vi "Test_Attribute.vi"() -> ()   [LabVIEW 2013]
uses:
  source/Serializer.INI/Serializer.PlainText.INI.lvclass
  source/Serializer/Serializer.lvclass
panel:
  out "String-formatted Value 2":string
  out "String-formatted Value":string
  out "String":string
  out "data":T1
  out "error out":errorcluster
  out "Section Attributes":variant
  out "Value":variant
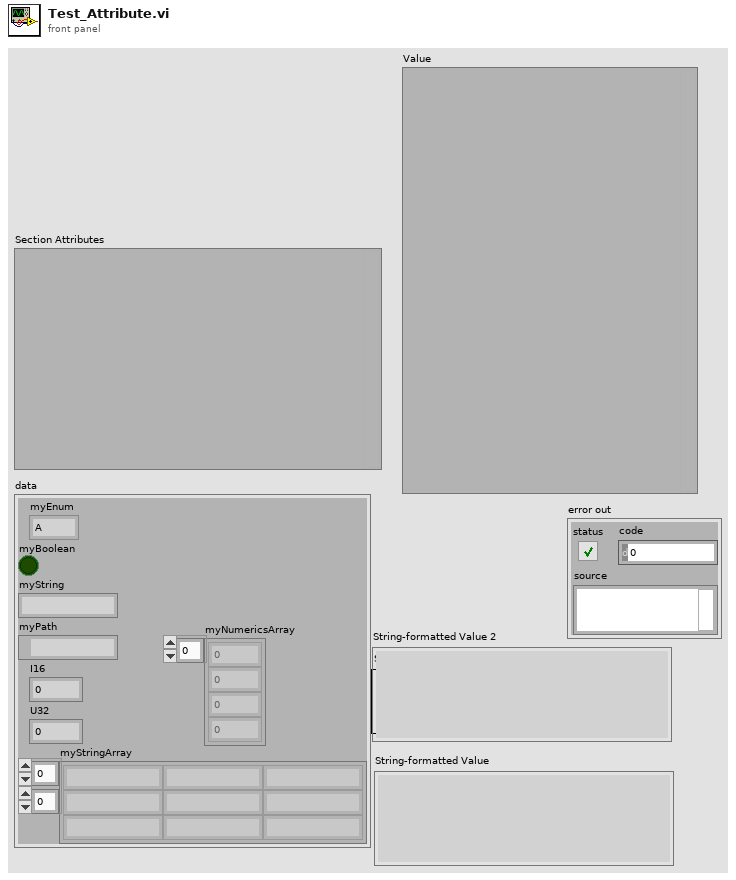
[diagram p1: front panel]
types:
  T1 = cluster{"myEnum":enum16{"A", "B", "C", "D"}, "myBoolean":bool, "myString":string, "myPath":path, "I16":i16, "U32":cdb, "myStringArray":string[][], "myNumericsArray":dbl[]}
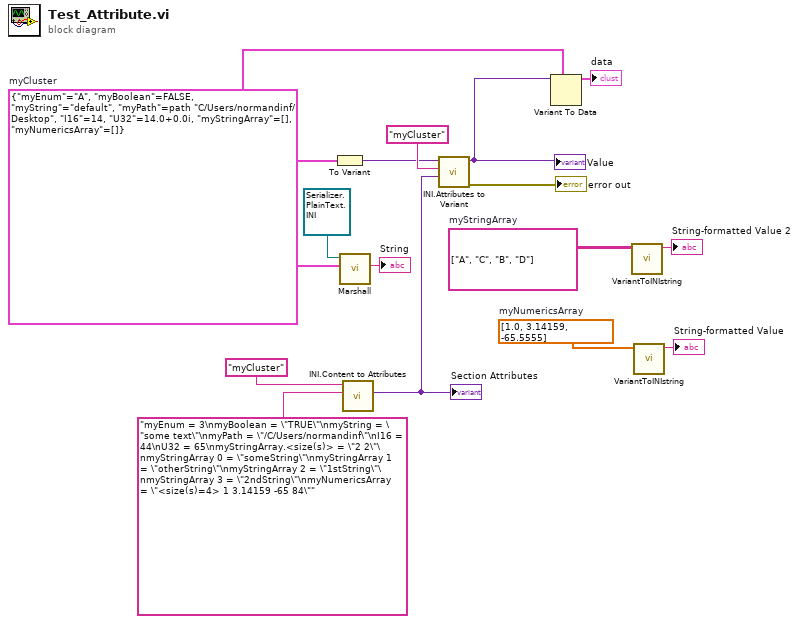
[diagram p0: block diagram]
diagram:
  w1 = string[][] [["A", "C"], ["B", "D"]]  # myStringArray
  w4 = dbl[] [1.0, 3.14159, -65.5555]  # myNumericsArray
  w6 = T1 {"myEnum"=enum."A", "myBoolean"=FALSE, "myString"="default", "myPath"=path "C:/Users/normandinf/Desktop", "I16"=14, "U32"=14.0+0.0i, "myStringArray"=[], "myNumericsArray"=[]}  # myCluster
  n1 = To Variant(anything=w6) -> (Variant=w11:variant)
  n2 = call "Marshall.vi"("Variant"=w6, "Serializer in"=refnum<class "Serializer.PlainText.INI.lvclass"> refnum ("Serializer.PlainText.INI.lvclass")) -> ("String"=→"String":string)  [unwired: 7 in, 2 out]
  n3 = call "INI.Content to Attributes.vi"("Content"="myEnum = 3\nmyBoolean = \"TRUE\"\nmyString = \"some text\"\nmyPath = \"/C/Users/normandinf\"\nI16 = 44\nU32 = 65\nmyStringArray.<size(s)> = \"2 2\"\nmyStringArray 0 = \"someString\"\nmyStringArray 1 = \"otherString\"\nmyStringArray 2 = \"1stString\"\nmyStringArray 3 = \"2ndString\"\nmyNumericsArray = \"<size(s)=4> 1 3.14159 -65 84\"", "Section Name"="myCluster" ("Content")) -> ("Section Attributes"=w15:variant)  [unwired: 9 in]
  "Section Attributes" <- w15
  n4 = call "INI.Attributes to Variant.vi"("Section Attribute"=w15, "Data Name"="myCluster" ("Content"), "Datatype"=w11) -> ("error out"=→"error out":errorcluster, "Variant"=w9:variant)  [unwired: 7 in]
  "Value" <- w9
  n5 = Variant To Data(type=w6, Variant=w9) -> (data=→"data":T1)  [unwired: 1 in, 1 out]
  n6 = call "VariantToINIstring.vi"("Variant-formatted Value"=w1) -> ("String-formatted Value"=→"String-formatted Value 2":string)  [unwired: 10 in]
  n7 = call "VariantToINIstring.vi"("Variant-formatted Value"=w4) -> ("String-formatted Value"=→"String-formatted Value":string)  [unwired: 10 in]
